vi "SetGain.vi"(8 "error in (no error)":errorcluster, 10 "Arg":string, 11 "ThorLabsCsCamera in":refnum<class "ThorLabsCsCamera.lvclass">) -> (0 "error out":errorcluster, 2 "setValue out":dbl, 3 "ThorLabsCsCamera out":refnum<class "ThorLabsCsCamera.lvclass">)   [LabVIEW 2020, in "ThorLabsCsCamera.lvclass"]
uses:
  ThorLabsCsCamera.lvclass
  ThorLabsCsCamera.lvclass/ThorLabsCsCamera.ctl
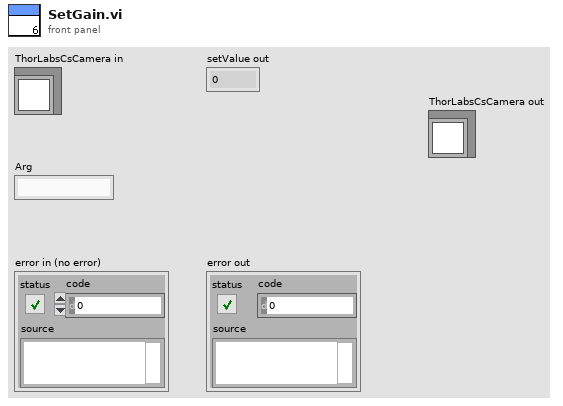
[diagram p1: front panel]
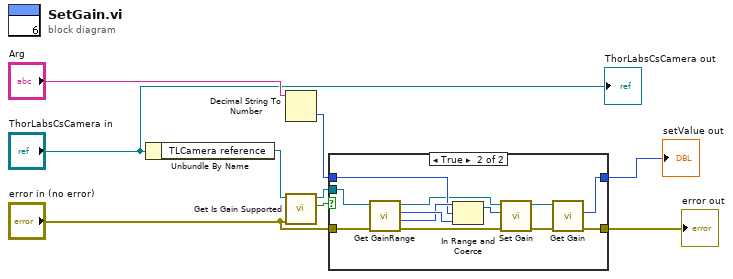
[diagram p0: block diagram]
diagram:
  n1 = Unbundle By Name("ThorLabsCsCamera in") -> ("TLCamera reference"=w4:refnum<k24>)
  n2 = Decimal String To Number(string="Arg") -> (number=w5:i32)  [unwired: 2 in, 1 out]
  n3 = call "Get Is Gain Supported.vi"("error in (no error)"="error in (no error)", "TLCamera reference in"=w4) -> ("Is Gain Supported?"=w2:bool, "TLCamera reference out"=w1:refnum<k24>)  [unwired: 7 in, 1 out]
  n4 = case shown="True" w2 {
    tunnel: [w10 w22] -> w7
    tunnel: [w11 w20] -> w6
    tunnel: w5 -> [w10 w17]
    tunnel: w1 -> [_ w13]
    tunnel: "error in (no error)" -> [w11 w12]
    frame False {
    }
    frame True {
      n5 = call "Get GainRange.vi"("error in (no error)"=w12, "TLCamera reference in"=w13) -> ("error out"=w14:errorcluster, "Maximum"=w18:u32, "Minimum"=w19:u32, "TLCamera reference out"=w15:refnum<k24>)  [unwired: 6 in]
      n6 = In Range and Coerce(upper limit=w18, x=w17, lower limit=w19) -> (coerced(x)=w16:u32)  [unwired: 1 out]
      n7 = call "Set Gain.vi"("error in (no error)"=w14, "Gain"=w16, "TLCamera reference in"=w15) -> ("error out"=w21:errorcluster, "TLCamera reference out"=w23:refnum<k24>)  [unwired: 7 in]
      n8 = call "Get Gain.vi"("error in (no error)"=w21, "TLCamera reference in"=w23) -> ("error out"=w20:errorcluster, "Gain"=w22:u32)  [unwired: 7 in, 1 out]
    }
  }
  "setValue out" <- w7
  "error out" <- w6
  "ThorLabsCsCamera out" <- "ThorLabsCsCamera in"
